vi "Downsample1D.vi"(9 "Avg N":i32, 11 "Array In":dbl[](array[numeric])) -> (3 "Array Out":dbl[](array[numeric]))   [LabVIEW 2013]
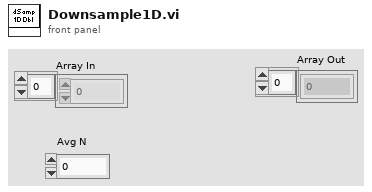
[diagram p1: front panel]
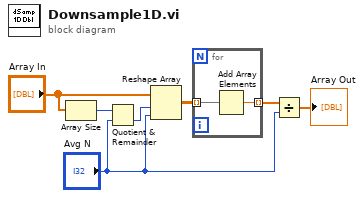
[diagram p0: block diagram]
diagram:
  n1 = Array Size(array="Array In") -> (size(s)=w1:i32)
  n2 = Quotient & Remainder(x=w1, y="Avg N") -> (floor(x/y)=w3:i32)  [unwired: 1 out]
  n3 = Reshape Array("Array In", w3, "Avg N") -> (w4:dbl[][])
  n4 = for {
    tunnel: w4 -> [w9] mode=indexing
    tunnel: [w8] -> w2 mode=indexing
    n5 = Add Array Elements(numeric array=w9) -> (sum=w8:dbl)
  }
  n6 = Divide(x=w2, y="Avg N") -> (x/y=→"Array Out":dbl[])
